vi "20181106_2.vi"() -> ()   [LabVIEW 2017]
panel:
  out "Gauge":dbl(knob) scale=0.0..10.0
  out "Total":i32
  out "floor(x/y)":i32
  in  "stop":bool
  out "min":dbl(knob) scale=0.0..10.0
  out "hr":dbl(knob) scale=0.0..10.0
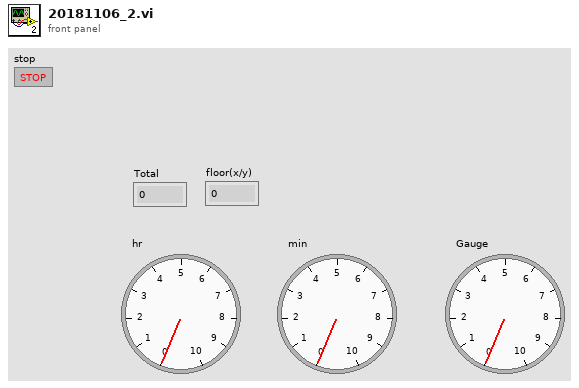
[diagram p1: front panel]
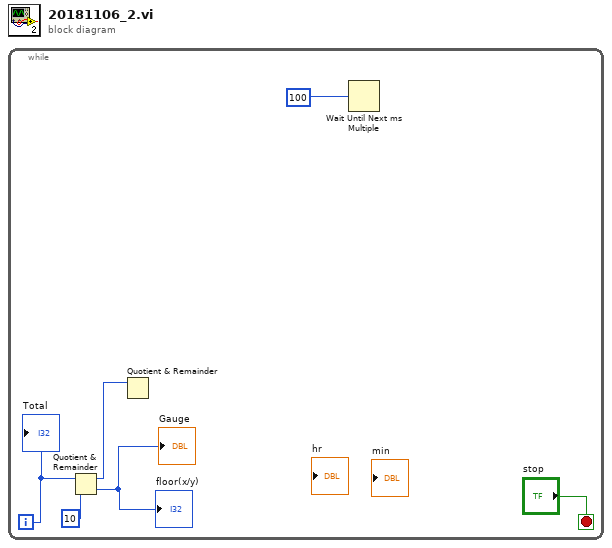
[diagram p0: block diagram]
diagram:
  n1 = while {
    i -> [w5]
    stop <- "stop" stop-if-true
    n2 = Quotient & Remainder(x=w5, y=10) -> (x-y*floor(x/y)=w1:i32, floor(x/y)=→"floor(x/y)" →"Gauge":i32)
    n3 = Quotient & Remainder(x=w1) -> ()  [unwired: 1 in, 2 out]
    n4 = Wait Until Next ms Multiple(millisecond multiple=100) -> ()  [unwired: 1 out]
    "Total" <- w5
  }
